vi "Format.vi"(8 "errin1":errorcluster caption="entrée d'erreur (pas d'erreur)", 11 "read buffer en entrée":string) -> (0 "errout":errorcluster caption="sortie d'erreur", 2 "VResult":string, 3 "TResult":string)   [LabVIEW 2020]
panel:
  in  "errin2":errorcluster caption="entrée d'erreur (pas d'erreur)"
  out "errout2":errorcluster caption="sortie d'erreur"
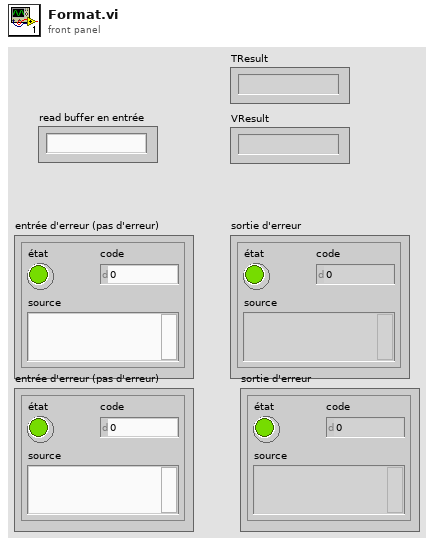
[diagram p1: front panel]
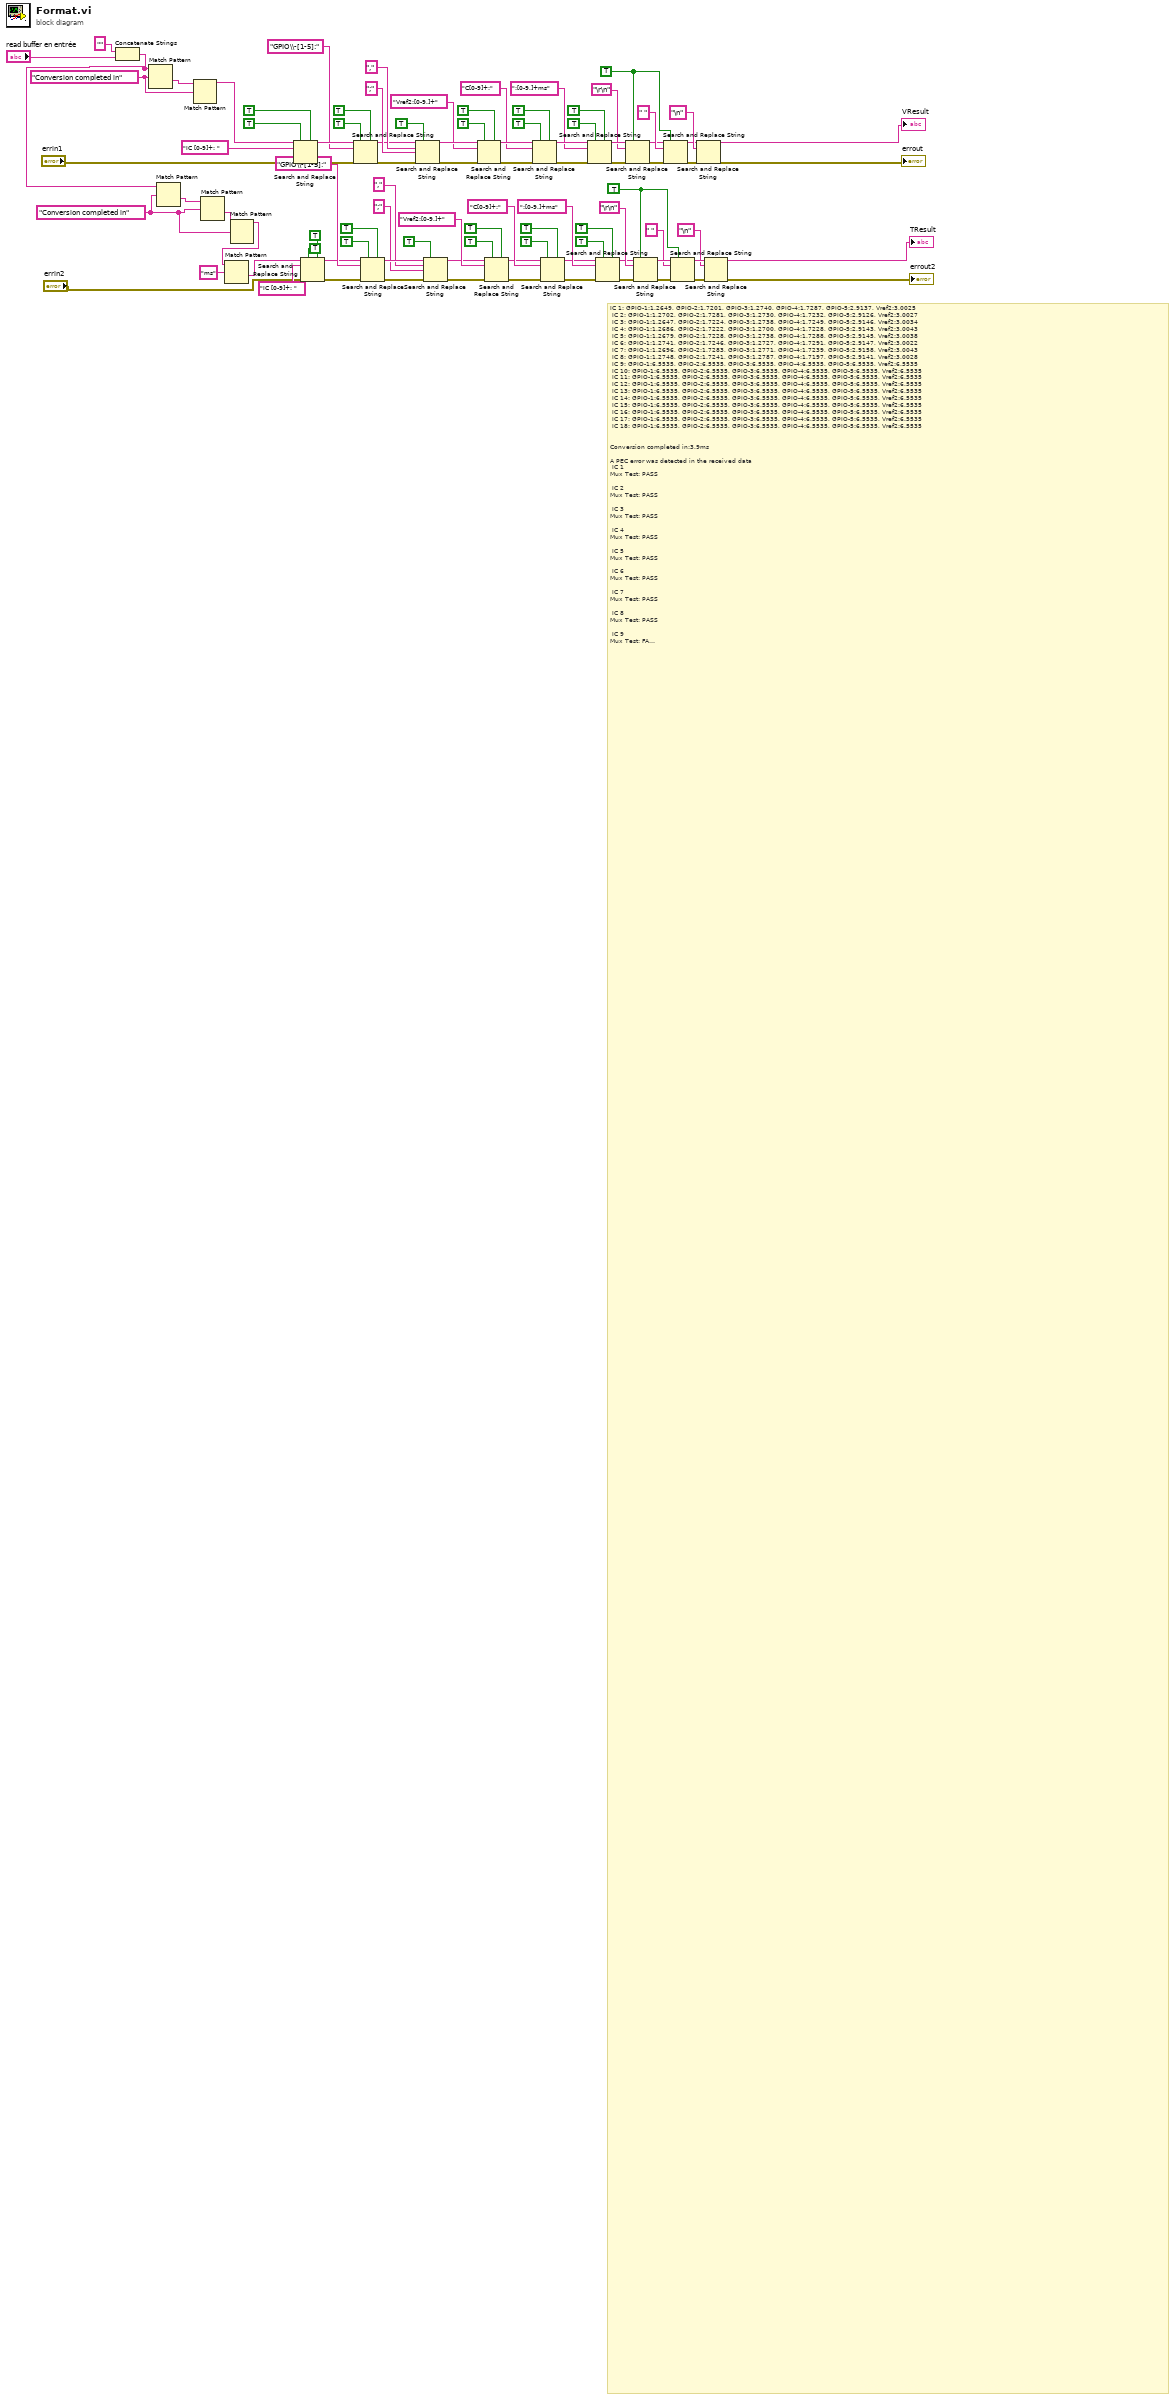
[diagram p0: block diagram]
diagram:
  w5 = "Conversion completed in" ("expression régulière")
  w26 = TRUE ("tout remplacer ? (F)")
  w83 = "Conversion completed in" ("expression régulière")
  w72 = TRUE ("tout remplacer ? (F)")
  # "IC 1: GPIO-1:1.2649, GPIO-2:1.7201, GPIO-3:1.2740, GPIO-4:1.7287, GPIO-5:2.9137, Vref2:3.0025\n IC 2: GPIO-1:1.2702, GPIO-2:1.7281, GPIO-3:1.2730, GPIO-4:1.7232, GPIO-5:2.9126, Vref2:3.0027\n IC 3: GPIO-1:1.2647, GPIO-2:1.7224, GPIO-3:1.2738, GPIO-4:1.7249, GPIO-5:2.9146, Vref2:3.0034\n IC 4: GPIO-1:1.2686, GPIO-2:1.7222, GPIO-3:1.2700, GPIO-4:1.7228, GPIO-5:2.9143, Vref2:3.0043\n IC 5: GPIO-1:1.2679, GPIO-2:1.7228, GPIO-3:1.2738, GPIO-4:1.7288, GPIO-5:2.9145, Vref2:3.0038\n IC 6: GPIO-1:1.2741, GPIO-2:1.7246, GPIO-3:1.2727, GPIO-4:1.7291, GPIO-5:2.9147, Vref2:3.0022\n IC 7: GPIO-1:1.2696, GPIO-2:1.7283, GPIO-3:1.2771, GPIO-4:1.7239, GPIO-5:2.9158, Vref2:3.0043\n IC 8: GPIO-1:1.2748, GPIO-2:1.7241, GPIO-3:1.2787, GPIO-4:1.7197, GPIO-5:2.9141, Vref2:3.0028\n IC 9: GPIO-1:6.5535, GPIO-2:6.5535, GPIO-3:6.5535, GPIO-4:6.5535, GPIO-5:6.5535, Vref2:6.5535\n IC 10: GPIO-1:6.5535, GPIO-2:6.5535, GPIO-3:6.5535, GPIO-4:6.5535, GPIO-5:6.5535, Vref2:6.5535\n IC 11: GPIO-1:6.5535, GPIO-2:6.5535, GPIO-3:6.5535, GPIO-4:6.5535, GPIO-5:6.5535, Vref2:6.5535\n IC 12: GPIO-1:6.5535, GPIO-2:6.5535, GPIO-3:6.5535, GPIO-4:6.5535, GPIO-5:6.5535, Vref2:6.5535\n IC 13: GPIO-1:6.5535, GPIO-2:6.5535, GPIO-3:6.5535, GPIO-4:6.5535, GPIO-5:6.5535, Vref2:6.5535\n IC 14: GPIO-1:6.5535, GPIO-2:6.5535, GPIO-3:6.5535, GPIO-4:6.5535, GPIO-5:6.5535, Vref2:6.5535\n IC 15: GPIO-1:6.5535, GPIO-2:6.5535, GPIO-3:6.5535, GPIO-4:6.5535, GPIO-5:6.5535, Vref2:6.5535\n IC 16: GPIO-1:6.5535, GPIO-2:6.5535, GPIO-3:6.5535, GPIO-4:6.5535, GPIO-5:6.5535, Vref2:6.5535\n IC 17: GPIO-1:6.5535, GPIO-2:6.5535, GPIO-3:6.5535, GPIO-4:6.5535, GPIO-5:6.5535, Vref2:6.5535\n IC 18: GPIO-1:6.5535, GPIO-2:6.5535, GPIO-3:6.5535, GPIO-4:6.5535, GPIO-5:6.5535, Vref2:6.5535\n\n\nConversion completed in:3.9ms \n\nA PEC error was detected in the received data\n IC 1\nMux Test: PASS \n\n IC 2\nMux Test: PASS \n\n IC 3\nMux Test: PASS \n\n IC 4\nMux Test: PASS \n\n IC 5\nMux Test: PASS \n\n IC 6\nMux Test: PASS \n\n IC 7\nMux Test: PASS \n\n IC 8\nMux Test: PASS \n\n IC 9\nMux Test: FAIL \n\n IC 10\nMux Test: FAIL \n\n IC 11\nMux Test: FAIL \n\n IC 12\nMux Test: FAIL \n\n IC 13\nMux Test: FAIL \n\n IC 14\nMux Test: FAIL \n\n IC 15\nMux Test: FAIL \n\n IC 16\nMux Test: FAIL \n\n IC 17\nMux Test: FAIL \n\n IC 18\nMux Test: FAIL \n\nConversion completed in:6.1ms \n\n IC 1:  C1:3.8925, C2:3.8936, C3:3.8932, C4:3.8937, C5:3.8930, C6:3.8926, C7:3.8923, C8:3.8921, C9:3.8911, C10:3.8913, C11:3.8919, C12:3.8918,\n IC 2:  C1:3.8922, C2:3.8914, C3:3.8913, C4:3.8913, C5:3.8903, C6:3.8911, C7:3.8907, C8:3.8906, C9:3.8898, C10:3.8898, C11:3.8902, C12:3.8911,\n IC 3:  C1:3.8922, C2:3.8924, C3:3.8929, C4:3.8927, C5:3.8903, C6:3.8915, C7:3.8924, C8:3.8930, C9:3.8909, C10:3.8933, C11:3.8918, C12:3.8932,\n IC 4:  C1:3.8940, C2:3.8915, C3:3.8915, C4:3.8928, C5:3.8926, C6:3.8925, C7:3.8917, C8:3.8913, C9:3.8903, C10:3.8913, C11:3.8895, C12:3.8915,\n IC 5:  C1:3.8926, C2:3.8911, C3:3.8902, C4:3.8927, C5:3.8914, C6:3.8918, C7:3.8942, C8:3.8935, C9:3.8925, C10:3.8923, C11:3.8917, C12:3.8928,\n IC 6:  C1:3.8920, C2:3.8926, C3:3.8931, C4:3.8929, C5:3.8924, C6:3.8929, C7:3.8911, C8:3.8920, C9:3.8904, C10:3.8927, C11:3.8919, C12:3.8914,\n IC 7:  C1:3.8935, C2:3.8921, C3:3.8931, C4:3.8940, C5:3.8934, C6:3.8925, C7:3.8928, C8:3.8912, C9:3.8927, C10:3.8912, C11:3.8920, C12:3.8924,\n IC 8:  C1:3.8927, C2:3.8926, C3:3.8930, C4:3.8887, C5:3.8915, C6:3.8925, C7:3.8899, C8:3.8921, C9:3.8914, C10:3.8919, C11:3.8911, C12:3.8910,\n IC 9:  C1:6.5535, C2:6.5535, C3:6.5535, C4:6.5535, C5:6.5535, C6:6.5535, C7:6.5535, C8:6.5535, C9:6.5535, C10:6.5535, C11:6.5535, C12:6.5535,\n IC 10:  C1:6.5535, C2:6.5535, C3:6.5535, C4:6.5535, C5:6.5535, C6:6.5535, C7:6.5535, C8:6.5535, C9:6.5535, C10:6.5535, C11:6.5535, C12:6.5535,\n IC 11:  C1:6.5535, C2:6.5535, C3:6.5535, C4:6.5535, C5:6.5535, C6:6.5535, C7:6.5535, C8:6.5535, C9:6.5535, C10:6.5535, C11:6.5535, C12:6.5535,\n IC 12:  C1:6.5535, C2:6.5535, C3:6.5535, C4:6.5535, C5:6.5535, C6:6.5535, C7:6.5535, C8:6.5535, C9:6.5535, C10:6.5535, C11:6.5535, C12:6.5535,\n IC 13:  C1:6.5535, C2:6.5535, C3:6.5535, C4:6.5535, C5:6.5535, C6:6.5535, C7:6.5535, C8:6.5535, C9:6.5535, C10:6.5535, C11:6.5535, C12:6.5535,\n IC 14:  C1:6.5535, C2:6.5535, C3:6.5535, C4:6.5535, C5:6.5535, C6:6.5535, C7:6.5535, C8:6.5535, C9:6.5535, C10:6.5535, C11:6.5535, C12:6.5535,\n IC 15:  C1:6.5535, C2:6.5535, C3:6.5535, C4:6.5535, C5:6.5535, C6:6.5535, C7:6.5535, C8:6.5535, C9:6.5535, C10:6.5535, C11:6.5535, C12:6.5535,\n IC 16:  C1:6.5535, C2:6.5535, C3:6.5535, C4:6.5535, C5:6.5535, C6:6.5535, C7:6.5535, C8:6.5535, C9:6.5535, C10:6.5535, C11:6.5535, C12:6.5535,\n IC 17:  C1:6.5535, C2:6.5535, C3:6.5535, C4:6.5535, C5:6.5535, C6:6.5535, C7:6.5535, C8:6.5535, C9:6.5535, C10:6.5535, C11:6.5535, C12:6.5535,\n IC 18:  C1:6.5535, C2:6.5535, C3:6.5535, C4:6.5535, C5:6.5535, C6:6.5535, C7:6.5535, C8:6.5535, C9:6.5535, C10:6.5535, C11:6.5535, C12:6.5535,\n\n\nConversion completed in:6.0ms \n\n IC 1: GPIO-1:1.2649, GPIO-2:1.7200, GPIO-3:1.2741, GPIO-4:1.7288, GPIO-5:2.9137, Vref2:3.0026\n IC 2: GPIO-1:1.2707, GPIO-2:1.7282, GPIO-3:1.2734, GPIO-4:1.7232, GPIO-5:2.9124, Vref2:3.0028\n IC 3: GPIO-1:1.2647, GPIO-2:1.7223, GPIO-3:1.2737, GPIO-4:1.7247, GPIO-5:2.9147, Vref2:3.0033\n IC 4: GPIO-1:1.2686, GPIO-2:1.7220, GPIO-3:1.2697, GPIO-4:1.7228, GPIO-5:2.9141, Vref2:3.0044\n IC 5: GPIO-1:1.2680, GPIO-2:1.7229, GPIO-3:1.2740, GPIO-4:1.7288, GPIO-5:2.9147, Vref2:3.0036\n IC 6: GPIO-1:1.2742, GPIO-2:1.7245, GPIO-3:1.2726, GPIO-4:1.7291, GPIO-5:2.9147, Vref2:3.0021\n IC 7: GPIO-1:1.2696, GPIO-2:1.7284, GPIO-3:1.2769, GPIO-4:1.7239, GPIO-5:2.9158, Vref2:3.0040\n IC 8: GPIO-1:1.2749, GPIO-2:1.7242, GPIO-3:1.2786, GPIO-4:1.7199, GPIO-5:2.9141, Vref2:3.0029\n IC 9: GPIO-1:6.5535, GPIO-2:6.5535, GPIO-3:6.5535, GPIO-4:6.5535, GPIO-5:6.5535, Vref2:6.5535\n IC 10: GPIO-1:6.5535, GPIO-2:6.5535, GPIO-3:6.5535, GPIO-4:6.5535, GPIO-5:6.5535, Vref2:6.5535\n IC 11: GPIO-1:6.5535, GPIO-2:6.5535, GPIO-3:6.5535, GPIO-4:6.5535, GPIO-5:6.5535, Vref2:6.5535\n IC 12: GPIO-1:6.5535, GPIO-2:6.5535, GPIO-3:6.5535, GPIO-4:6.5535, GPIO-5:6.5535, Vref2:6.5535\n IC 13: GPIO-1:6.5535, GPIO-2:6.5535, GPIO-3:6.5535, GPIO-4:6.5535, GPIO-5:6.5535, Vref2:6.5535\n IC 14: GPIO-1:6.5535, GPIO-2:6.5535, GPIO-3:6.5535, GPIO-4:6.5535, GPIO-5:6.5535, Vref2:6.5535\n IC 15: GPIO-1:6.5535, GPIO-2:6.5535, GPIO-3:6.5535, GPIO-4:6.5535, GPIO-5:6.5535, Vref2:6.5535\n IC 16: GPIO-1:6.5535, GPIO-2:6.5535, GPIO-3:6.5535, GPIO-4:6.5535, GPIO-5:6.5535, Vref2:6.5535\n IC 17: GPIO-1:6.5535, GPIO-2:6.5535, GPIO-3:6.5535, GPIO-4:6.5535, GPIO-5:6.5535, Vref2:6.5535\n IC 18: GPIO-1:6.5535, GPIO-2:6.5535, GPIO-3:6.5535, GPIO-4:6.5535, GPIO-5:6.5535, Vref2:6.5535\n\n\nConversion completed in:4.0ms \n\nA PEC error was detected in the received data\n IC 1\nMux Test: PASS \n\n IC 2\nMux Test: PASS \n\n IC 3\nMux Test: PASS \n\n IC 4\nMux Test: PASS \n\n IC 5\nMux Test: PASS \n\n IC 6\nMux Test: PASS \n\n IC 7\nMux Test: PASS \n\n IC 8\nMux Test: PASS \n\n IC 9\nMux Test: FAIL \n\n IC 10\nMux Test: FAIL \n\n IC 11\nMux Test: FAIL \n\n IC 12\nMux Test: FAIL \n\n IC 13\nMux Test: FAIL \n\n IC 14\nMux Test: FAIL \n\n IC 15\nMux Test: FAIL \n\n IC 16\nMux Test: FAIL \n\n IC 17\nMux Test: FAIL \n\n IC 18\nMux Test: FAIL \n\nConversion completed in:6.0ms \n\n IC 1:  C1:3.8924, C2:3.8937, C3:3.8933, C4:3.8937, C5:3.8928, C6:3.8"
  n1 = Concatenate Strings("", "read buffer en entrée") -> (w7:string)
  n2 = Match Pattern ("Rechercher une expression")(string=w7, regular expression=w83) -> (after substring=w82:string)  [unwired: 1 in, 3 out]
  n3 = Match Pattern ("Rechercher une expression")(string=w7, regular expression=w5) -> (after substring=w17:string)  [unwired: 1 in, 3 out]
  n4 = Match Pattern ("Rechercher une expression")(string=w82, regular expression=w83) -> (before substring=w93:string)  [unwired: 1 in, 3 out]
  n5 = Match Pattern ("Rechercher une expression")(string=w17, regular expression=w5) -> (after substring=w6:string)  [unwired: 1 in, 3 out]
  n6 = Match Pattern ("Rechercher une expression")(string=w6, regular expression=w5) -> (before substring=w4:string)  [unwired: 1 in, 3 out]
  n7 = Match Pattern ("Rechercher une expression")(string=w4, regular expression="ms" ("expression régulière")) -> (after substring=w2:string)  [unwired: 1 in, 3 out]
  n8 = Search and Replace String ("Rechercher et remplacer une chaîne")(replace all?=TRUE ("tout remplacer ? (F)"), multiline?=TRUE ("multiligne ? (F)"), input string=w93, search string="IC [0-9]+: " ("chaîne recherchée"), error in="errin1") -> (result string=w56:string, error out=w84:errorcluster)  [unwired: 3 in, 2 out]
  n9 = Search and Replace String ("Rechercher et remplacer une chaîne")(replace all?=TRUE ("tout remplacer ? (F)"), multiline?=TRUE ("multiligne ? (F)"), input string=w2, search string="IC [0-9]+: " ("chaîne recherchée"), error in="errin2") -> (result string=w42:string, error out=w16:errorcluster)  [unwired: 3 in, 2 out]
  n10 = Search and Replace String ("Rechercher et remplacer une chaîne")(replace all?=TRUE ("tout remplacer ? (F)"), multiline?=TRUE ("multiligne ? (F)"), input string=w56, search string="GPIO\\-[1-5]:" ("chaîne recherchée"), error in=w84) -> (result string=w76:string, error out=w85:errorcluster)  [unwired: 3 in, 2 out]
  n11 = Search and Replace String ("Rechercher et remplacer une chaîne")(replace all?=TRUE ("tout remplacer ? (F)"), multiline?=TRUE ("multiligne ? (F)"), input string=w42, search string="GPIO\\-[1-5]:" ("chaîne recherchée"), error in=w16) -> (result string=w22:string, error out=w15:errorcluster)  [unwired: 3 in, 2 out]
  n12 = Search and Replace String ("Rechercher et remplacer une chaîne")(replace all?=TRUE ("tout remplacer ? (F)"), input string=w76, search string="," ("chaîne recherchée"), replace string=";" ("chaîne de remplacement (\"\")"), error in=w85) -> (result string=w77:string, error out=w86:errorcluster)  [unwired: 3 in, 2 out]
  n13 = Search and Replace String ("Rechercher et remplacer une chaîne")(replace all?=TRUE ("tout remplacer ? (F)"), input string=w22, search string="," ("chaîne recherchée"), replace string=";" ("chaîne de remplacement (\"\")"), error in=w15) -> (result string=w21:string, error out=w14:errorcluster)  [unwired: 3 in, 2 out]
  n14 = Search and Replace String ("Rechercher et remplacer une chaîne")(replace all?=TRUE ("tout remplacer ? (F)"), multiline?=TRUE ("multiligne ? (F)"), input string=w77, search string="Vref2:[0-9.]+" ("chaîne recherchée"), error in=w86) -> (result string=w63:string, error out=w87:errorcluster)  [unwired: 3 in, 2 out]
  n15 = Search and Replace String ("Rechercher et remplacer une chaîne")(replace all?=TRUE ("tout remplacer ? (F)"), multiline?=TRUE ("multiligne ? (F)"), input string=w21, search string="Vref2:[0-9.]+" ("chaîne recherchée"), error in=w14) -> (result string=w35:string, error out=w13:errorcluster)  [unwired: 3 in, 2 out]
  n16 = Search and Replace String ("Rechercher et remplacer une chaîne")(replace all?=TRUE ("tout remplacer ? (F)"), multiline?=TRUE ("multiligne ? (F)"), input string=w63, search string="C[0-9]+:" ("chaîne recherchée"), error in=w87) -> (result string=w65:string, error out=w88:errorcluster)  [unwired: 3 in, 2 out]
  n17 = Search and Replace String ("Rechercher et remplacer une chaîne")(replace all?=TRUE ("tout remplacer ? (F)"), multiline?=TRUE ("multiligne ? (F)"), input string=w35, search string="C[0-9]+:" ("chaîne recherchée"), error in=w13) -> (result string=w33:string, error out=w12:errorcluster)  [unwired: 3 in, 2 out]
  n18 = Search and Replace String ("Rechercher et remplacer une chaîne")(replace all?=TRUE ("tout remplacer ? (F)"), multiline?=TRUE ("multiligne ? (F)"), input string=w65, search string=":[0-9.]+ms" ("chaîne recherchée"), error in=w88) -> (result string=w69:string, error out=w89:errorcluster)  [unwired: 3 in, 2 out]
  n19 = Search and Replace String ("Rechercher et remplacer une chaîne")(replace all?=TRUE ("tout remplacer ? (F)"), multiline?=TRUE ("multiligne ? (F)"), input string=w33, search string=":[0-9.]+ms" ("chaîne recherchée"), error in=w12) -> (result string=w29:string, error out=w11:errorcluster)  [unwired: 3 in, 2 out]
  n20 = Search and Replace String ("Rechercher et remplacer une chaîne")(replace all?=w72, input string=w69, search string="\r\n", error in=w89) -> (result string=w70:string, error out=w91:errorcluster)  [unwired: 4 in, 2 out]
  n21 = Search and Replace String ("Rechercher et remplacer une chaîne")(replace all?=w26, input string=w29, search string="\r\n", error in=w11) -> (result string=w28:string, error out=w9:errorcluster)  [unwired: 4 in, 2 out]
  n22 = Search and Replace String ("Rechercher et remplacer une chaîne")(replace all?=w72, input string=w70, search string=" " ("chaîne recherchée"), error in=w91) -> (result string=w73:string, error out=w90:errorcluster)  [unwired: 4 in, 2 out]
  n23 = Search and Replace String ("Rechercher et remplacer une chaîne")(replace all?=w26, input string=w28, search string=" " ("chaîne recherchée"), error in=w9) -> (result string=w25:string, error out=w10:errorcluster)  [unwired: 4 in, 2 out]
  n24 = Search and Replace String ("Rechercher et remplacer une chaîne")(input string=w73, search string="\n" ("chaîne recherchée"), error in=w90) -> (result string=→"VResult":string, error out=→"errout":errorcluster)  [unwired: 5 in, 2 out]
  n25 = Search and Replace String ("Rechercher et remplacer une chaîne")(input string=w25, search string="\n" ("chaîne recherchée"), error in=w10) -> (result string=→"TResult":string, error out=→"errout2":errorcluster)  [unwired: 5 in, 2 out]
